vi "Get UDP Reference.vi"(8 "error in (no error)":errorcluster, 11 "Assert UID":string) -> (0 "error out":errorcluster, 2 "UDP Reference":refnum<k16>)   [LabVIEW 2016, in "Assert API Components.lvlib" / "Log Assert Core.lvlib"]
uses:
  Log Assert Core.lvlib
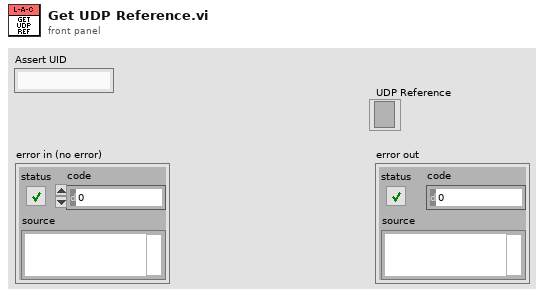
[diagram p1: front panel]
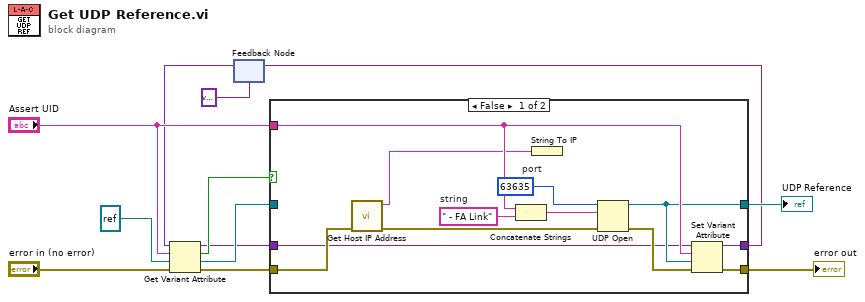
[diagram p0: block diagram]
diagram:
  n1 = feedback #1(variant) -> (w8:variant)
  n2 = Get Variant Attribute(Variant=w8, name="Assert UID", default value (empty Variant)=refnum<k16> refnum ("UDP Reference"), error in="error in (no error)") -> (duplicate Variant=w2:variant, found=w5:bool, value=w4:refnum<k16>, error out=w6:errorcluster)
  n3 = case shown="False" w5 {
    tunnel: [w20 w27] -> w11
    tunnel: w6 -> [w19 w27]
    tunnel: "Assert UID" -> [w18 _]
    tunnel: w4 -> [_ w26]
    tunnel: [w17 w26] -> w7
    tunnel: [w16 w25] -> w1
    tunnel: w2 -> [w15 w25]
    frame False {
      w22 = " - FA Link"  # string
      w23 = u16 63635  # port
      n4 = call "Get Host IP Address.vi"("error in (no error)"=w19) -> ("error out"=w14:errorcluster, "Host IP Address"=w13:string)  [unwired: 9 in]
      n5 = Concatenate Strings(w18, w22) -> (w21:string)
      n6 = String To IP(1:w13) -> ()  [unwired: 1 out]
      n7 = UDP Open(8:w14, 10:w21, 11:w23) -> (port=w17:refnum<k16>, 0:w24:errorcluster)  [unwired: 2 in, 1 out]
      n8 = Set Variant Attribute(Variant=w15, name=w18, value=w17, error in=w24) -> (Variant out=w16:variant, error out=w20:errorcluster)  [unwired: 1 out]
    }
    frame True {
    }
  }
  "error out" <- w11
  "UDP Reference" <- w7
  n9 = feedback-in #1(w1) -> ()
